vi "Is Recieve Ready.vi"(8 "error in (no error)":errorcluster, 10 "Points to read":i32, 11 "RP Instrument in":refnum<class "RP Instrument.lvclass">) -> (0 "error out":errorcluster, 1 "Points in buffer":i32, 2 "Recieve Ready":bool, 3 "RP Instrument out":refnum<class "RP Instrument.lvclass">)   [LabVIEW 2015, in "RP Instrument.lvclass"]
uses:
  RP Instrument.lvclass
  RP Status Offsets.ctl
  RP Instrument.lvclass/RP Instrument.ctl
  RP Communicator/RP Communicator.lvclass
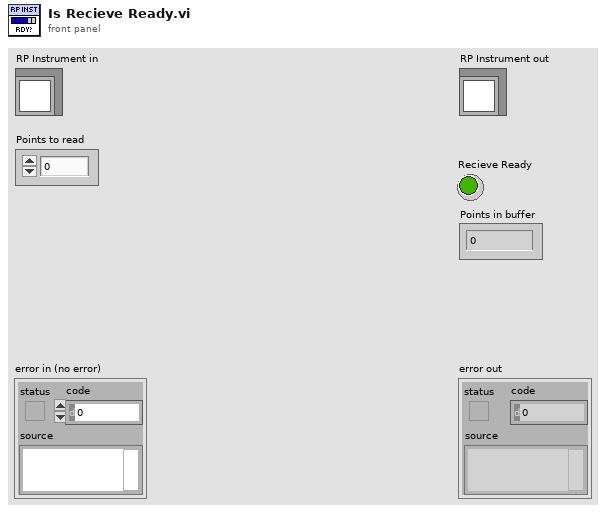
[diagram p1: front panel]
types:
  T1 = typedef "RP Status Offsets.ctl" = u16
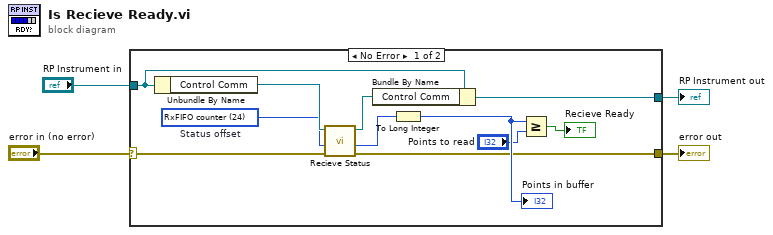
[diagram p0: block diagram]
diagram:
  n1 = case shown="No Error" "error in (no error)" {
    selector: "error in (no error)" -> [w7 w17]
    tunnel: [w6 w17] -> w3
    tunnel: [w9 w16] -> w1
    tunnel: "RP Instrument in" -> [w15 w16]
    frame No Error {
      w13 = T1 24 items=["Writer address"=0, "Record start position"=4, "Trig state etc."=8, "RxFIFO counter"=24, "TxFIFO counter"=28]  # Status offset
      n2 = Unbundle By Name(w15) -> ("Control Comm"=w14:refnum<class "RP Communicator.lvclass">)
      n3 = call-dynamic "Recieve Status.vi"("error in (no error)"=w7, "Status offset"=w13, "RP Communicator in"=w14) -> ("error out"=w6:errorcluster, "Status response"=w11:u32, "RP Communicator out"=w8:refnum<class "RP Communicator.lvclass">)  [unwired: 6 in]
      n4 = Bundle By Name(cluster=w15, "Control Comm"=w8) -> (w9:refnum<class "RP Instrument.lvclass">)
      n5 = To Long Integer(number=w11) -> (32bit integer=w12:i32)
      "Points in buffer" <- w12
      n6 = Greater Or Equal?(x=w12, y="Points to read") -> (x >= y?=→"Recieve Ready":bool)
    }
    frame Error {
    }
  }
  "error out" <- w3
  "RP Instrument out" <- w1
